vi "CorShowCohort.vi"(6 "error in (no error)":errorcluster, 7 "Group #":u8, 8 "Cohorts in":refnum<class "Cohort.lvclass">[](array[class]), 9 "Coh Panel in":refnum<vi>) -> (0 "error out":errorcluster, 2 "Cohort out":refnum<class "Cohort.lvclass">, 3 "Coh Panel out":refnum<vi>)   [LabVIEW 2012, in "Cohort.lvclass"]
uses:
  Cohort.lvclass
  CohortConfig.ctl
  UserControl/LeftPanel.ctl
  UserControl/ElectdPanel.ctl
  UserControl/ElectdTerminal.ctl
  Cohort.lvclass/Cohort.ctl
  StimulCtrls.lvlib
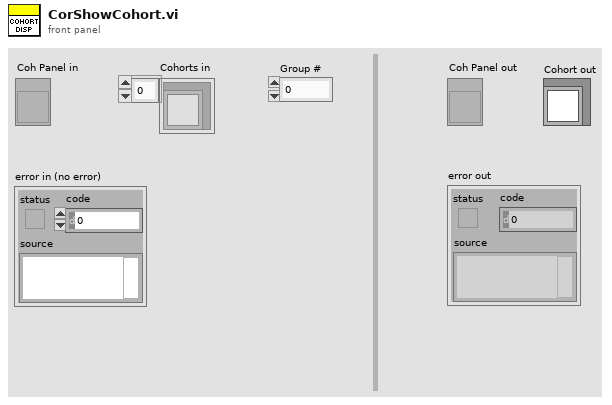
[diagram p1: front panel]
types:
  T1 = enum8{"Enabled", "Disabled", "Disabled and Grayed Out"}
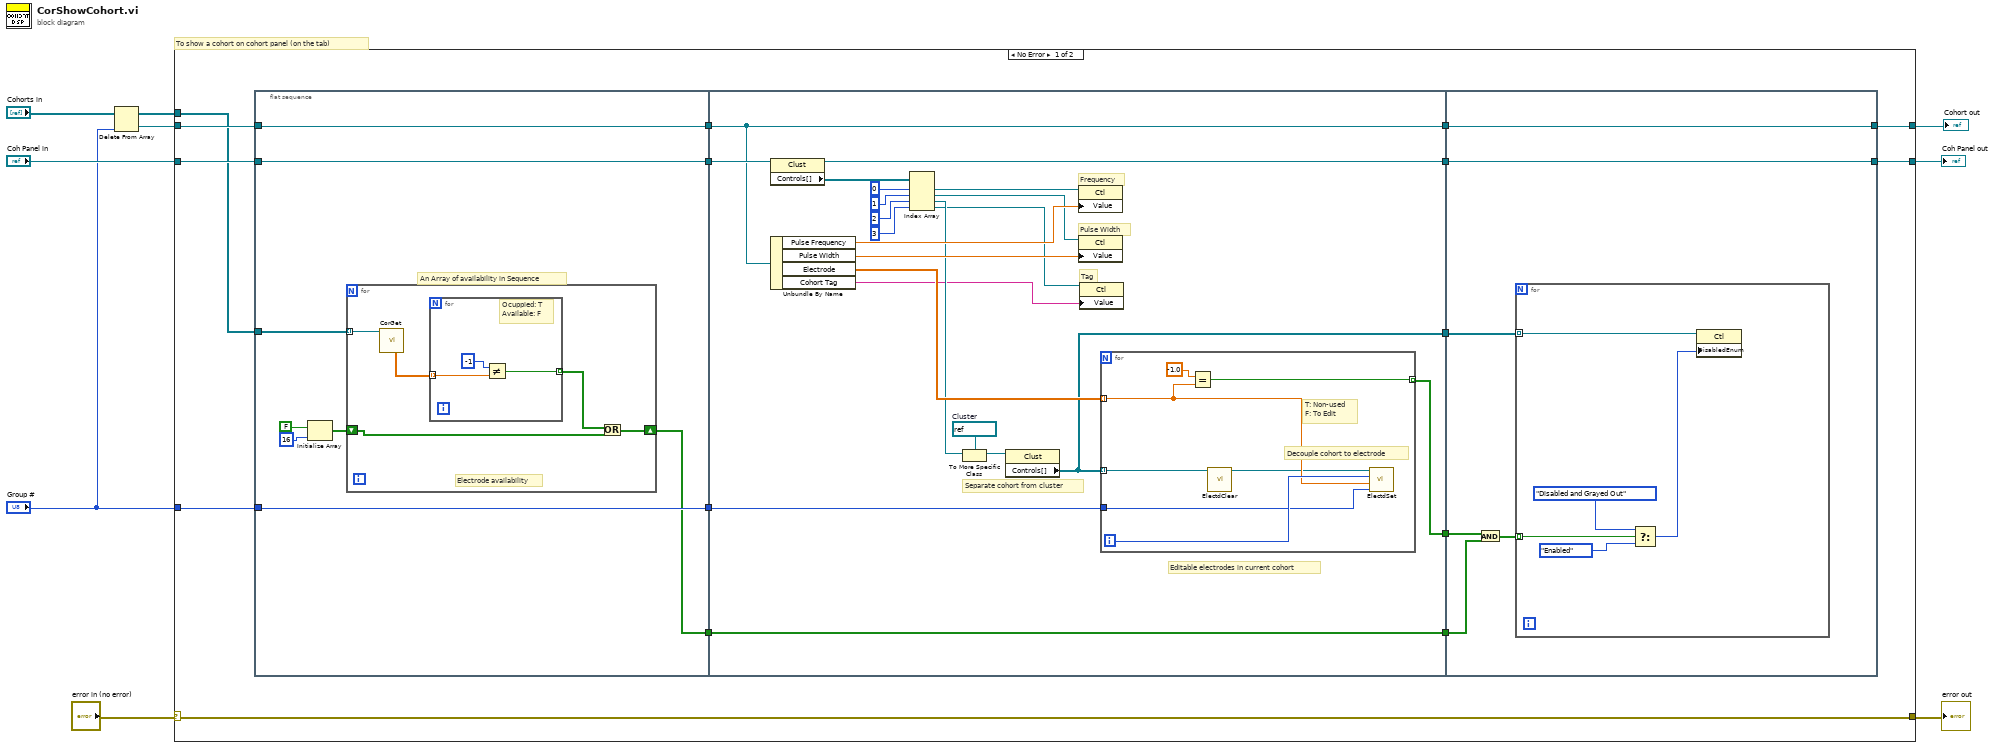
[diagram p0: block diagram]
diagram:
  # "To show a cohort on cohort panel (on the tab)"
  n1 = Delete From Array(array="Cohorts in", index="Group #") -> (deleted portion=w2:refnum<class "Cohort.lvclass">, array with subset deleted=w1:refnum<class "Cohort.lvclass">[])  [unwired: 1 in]
  n2 = case shown="No Error" "error in (no error)" {
    selector: "error in (no error)" -> [w25 w84]
    tunnel: [w25 w84] -> w8
    tunnel: [w24 w83] -> w7
    tunnel: "Group #" -> [w12 _]
    tunnel: "Coh Panel in" -> [w15 w83]
    tunnel: [w14 w82] -> w5
    tunnel: w2 -> [w11 w82]
    tunnel: w1 -> [w10 _]
    frame No Error {
      n3 = flat-sequence {
        tunnel: w12 -> [w30]
        tunnel: [w26] -> w23
        tunnel: [w30] -> w22
        tunnel: [w29] -> w18
        tunnel: [w28] -> w16
        tunnel: w15 -> [w28]
        tunnel: w10 -> [w27]
        tunnel: w11 -> [w26]
        tunnel: w23 -> [w45]
        tunnel: w22 -> [w50]
        tunnel: [w51] -> w21
        tunnel: [w49] -> w20
        tunnel: [w48] -> w19
        tunnel: w18 -> [w48]
        tunnel: [w47] -> w17
        tunnel: w16 -> [w46]
        tunnel: [w45] -> w13
        tunnel: [w76] -> w24
        tunnel: w21 -> [w76]
        tunnel: w20 -> [w75]
        tunnel: w19 -> [w74]
        tunnel: w17 -> [w72]
        tunnel: [w71] -> w14
        tunnel: w13 -> [w71]
        frame #0 {
          # "An Array of availability in Sequence"
          n4 = Initialize Array(FALSE, 16 ("dimension size")) -> (w33:bool[])
          n5 = for {
            tunnel: w27 -> [w38] mode=indexing
            shift-right: [w36] -> w29
            shift-left: w33 -> [w34]
            # "Electrode availability"
            n6 = call-dynamic "CorGet.vi"("Cohort in"=w38) -> ("Amplitude"=w37:sgl[])  [unwired: 6 in, 4 out]
            n7 = for {
              tunnel: w37 -> [w41] mode=indexing
              tunnel: [w39] -> w35 mode=indexing
              # "Ocuppied: T\nAvailable: F"
              n8 = Not Equal?(x=-1, y=w41) -> (x != y?=w39:bool)
            }
            n9 = Or(x=w35, y=w34) -> (x .or. y?=w36:bool[])
          }
        }
        frame #1 {
          w54 = refnum<vi> refnum  # Cluster
          # "Tag"
          # "Editable electrodes in current cohort"
          # "Separate cohort from cluster"
          # "Pulse Width"
          # "Frequency"
          n10 = property class="Clust"(reference=w46) -> (reference out=w51:refnum<vi>, "Controls[]"=w62:refnum<vi>[])  [unwired: 1 in, 1 out]
          n11 = Unbundle By Name(w45) -> ("Pulse Frequency"=w59:sgl, "Pulse Width"=w55:sgl, "Electrode"=w63:sgl[], "Cohort Tag"=w42:string)
          n12 = Index Array(array=w62, index #1=0 ("index"), index #2=1 ("index"), index #3=2 ("index"), index #4=3 ("index")) -> (element #1=w60:refnum<vi>, element #2=w56:refnum<vi>, element #3=w52:refnum<vi>, element #4=w43:refnum<vi>)
          n13 = To More Specific Class(target class=w54, reference=w52) -> (specific class reference=w53:refnum<vi>)  [unwired: 1 in, 1 out]
          n14 = property class="Clust"(reference=w53) -> ("Controls[]"=w47:refnum<vi>[])  [unwired: 1 in, 2 out]
          n15 = property class="Ctl"(reference=w60, "Value"=w59) -> ()  [unwired: 1 in, 2 out]
          n16 = property class="Ctl"(reference=w56, "Value"=w55) -> ()  [unwired: 1 in, 2 out]
          n17 = property class="Ctl"(reference=w43, "Value"=w42) -> ()  [unwired: 1 in, 2 out]
          n18 = for {
            tunnel: w63 -> [w68] mode=indexing
            tunnel: w47 -> [w65] mode=indexing
            tunnel: w50 -> [w69]
            tunnel: [w66] -> w49 mode=indexing
            i -> [w70]
            # "T: Non-used\nF: To Edit"
            # "Decouple cohort to electrode"
            n19 = Equal?(x=sgl -1.0, y=w68) -> (x = y?=w66:bool)
            n20 = call "ElectdClear.vi"("Electd in"=w65) -> ("Electd out"=w64:refnum<vi>)  [unwired: 10 in]
            n21 = call "ElectdSet.vi"("Group #"=w69, "Amplitude"=w68, "Index"=w70, "Electd Panel in"=w64) -> ()  [unwired: 7 in, 1 out]
          }
        }
        frame #2 {
          n22 = And(x=w75, y=w74) -> (x .and. y?=w73:bool[])
          n23 = for {
            tunnel: w72 -> [w81] mode=indexing
            tunnel: w73 -> [w80] mode=indexing
            n24 = Select(t=T1."Disabled and Grayed Out" ("Disabled"), s=w80, f=T1."Enabled" ("Disabled")) -> (s? t:f=w77:T1)
            n25 = property class="Ctl"(reference=w81, "DisabledEnum"=w77) -> ()  [unwired: 1 in, 2 out]
          }
        }
      }
    }
    frame Error {
    }
  }
  "error out" <- w8
  "Coh Panel out" <- w7
  "Cohort out" <- w5
